vi "Connect temp (SubIV).vi"(8 "Error In":errorcluster, 11 "Loop data In":T2={"Persistent"={"Last file"=path "", "Last user"="", "Users"=[]}, "Temp handle"={"Connected"=FALSE, "Temp ctrl"={"Gain (P)"=0.0, "Reset (I)"=0.0, "Rate (D)"=0.0, "Stabilization rate"=0.0, "Stabilization delta"=0.0, "Type"=enum."Lake Shore 325", "Custom temp ctrl"={"VISA resource name"=""}, "Lakeshore 325"={"VISA name"="", "Loop"=0, "Heater Range"=1, "Heater Resistance"=0, "Sample sensor"=0, "Fast sensor"=0, "Slow sensor"=0}, "Lakeshore 331"={"VISA name"="", "Loop"=1, "Heater Range"=0, "Sample sensor"=0, "Fast sensor"=0, "Slow sensor"=0}, "Lakeshore 332"={"VISA name"="", "Loop"=1, "Heater Range"=0, "Sample sensor"=0, "Fast sensor"=0, "Slow sensor"=0}, "Lakeshore 335"={"VISA name"="", "Loop"=1, "Sample sensor"=0, "Fast sensor"=0, "Slow sensor"=0, "Heater Range"=0, "Output mode"=enum."Off"}, "Lakeshore 336"={"VISA name"="", "Loop"=1, "Output mode"=enum."Off", "Max current"=0.0, "Heater resistance"=0, "Sample sensor"=0, "Slow sensor"=0, "Fast sensor"=1}}}, "Paths"={"Manual"=path "", "Settings"=path "", "Persistent"=path "", "Work dir."=path ""}, "Settings"={"MFIA"={"Address"="", "Use compensation"=TRUE, "Shut down gracefully"=FALSE}, "Temp ctrl"={"Gain (P)"=0.0, "Reset (I)"=0.0, "Rate (D)"=0.0, "Stabilization rate"=0.0, "Stabilization delta"=0.0, "Type"=enum."Lake Shore 325", "Custom temp ctrl"={"VISA resource name"=""}, "Lakeshore 325"={"VISA name"="", "Loop"=0, "Heater Range"=1, "Heater Resistance"=0, "Sample sensor"=0, "Fast sensor"=0, "Slow sensor"=0}, "Lakeshore 331"={"VISA name"="", "Loop"=1, "Heater Range"=0, "Sample sensor"=0, "Fast sensor"=0, "Slow sensor"=0}, "Lakeshore 332"={"VISA name"="", "Loop"=1, "Heater Range"=0, "Sample sensor"=0, "Fast sensor"=0, "Slow sensor"=0}, "Lakeshore 335"={"VISA name"="", "Loop"=1, "Sample sensor"=0, "Fast sensor"=0, "Slow sensor"=0, "Heater Range"=0, "Output mode"=enum."Off"}, "Lakeshore 336"={"VISA name"="", "Loop"=1, "Output mode"=enum."Off", "Max current"=0.0, "Heater resistance"=0, "Sample sensor"=0, "Slow sensor"=0, "Fast sensor"=1}}, "Source-meter"={"Type"=enum."Custom", "Custom source-meter"={"VISA resource name"=""}, "Keithley 2600"={"VISA name"="", "Ignore ID Query"=FALSE, "SMU"=enum."Channel A"}}, "Other"={"Enable OriginLab"=FALSE, "Reader mode"=FALSE, "Auto-save"=FALSE}, "Defaults"={"IV properties"={"T"=0.0, "Vstart"=-0.5, "Vstop"=0.5, "Vpoints"=10.0, "Settling"=0.01, "I limit"=0.1, "Log mapping"=FALSE, "Averaging"=0.0}, "CV properties"={"T"=0.0, "Vstart"=-0.5, "Vstop"=0.5, "Vpoints"=10.0, "Precision"=enum."Normal", "Test signal"=0.01, "Auto I range"=FALSE, "Test frequency"=100000.0, "I range"=-2.0, "V range"=10.0, "Log mapping"=FALSE, "Rel perm"=0.0, "Area"=0.0}, "DLTS properties"={"Tstart"=0.0, "Instant start"=FALSE, "Tstop"=0.0, "T rate"=0.0, "Test signal"=0.0, "Test frequency"=0.0, "Bandwidth"=0.0, "Averaging"=0.0, "Vbias"=0.0, "Vpulse"=0.0, "pulse length"=0.0, "Pulse 2"=FALSE, "Vpulse 2"=0.0, "pulse length 2"=0.0, "I range"=-2.0, "V range"=10.0, "Emission rate"=[], "Sampling rate"=0.0, "Acq. delay"=0.0}, "LDLTS properties"={"T"=0.0, "Test signal"=0.0, "Test frequency"=0.0, "Bandwidth"=0.0, "Averaging"=0.0, "Vbias"=0.0, "Vpulse"=0.0, "pulse length"=0.0, "Pulse 2"=FALSE, "Vpulse 2"=0.0, "pulse length 2"=0.0, "I range"=-2.0, "V range"=10.0, "Sampling rate"=0.0, "Acq. delay"=0.0, "Sampling time"=0.0}}}, "Software version"=0.0, "MFIA handle"={"ziHandle"={"handleValid"=FALSE, "Conn"=0, "Path Prefix"="", "Handle"=0, "Connected"=FALSE, "Clockbase(s)"=0.0}, "Selected device"="", "ziModHandle"={"handleValid"=FALSE, "Conn"=0, "ModHandle"=0, "moduleID"="", "Path Prefix"=""}}, "Source-meter handle"={"Connected"=FALSE, "Source-meter"={"Type"=enum."Keithley 2600", "Custom source-meter"={"VISA resource name"=""}, "Keithley 2600"={"VISA name"="", "Ignore ID Query"=FALSE, "SMU"=enum."Channel A"}}}} {"MFIA handle"."ziModHandle"."ModHandle" format="0x%08x"; "MFIA handle"."ziModHandle"."Conn" format="0x%08x"; "MFIA handle"."ziHandle"."Handle" format="0x%08x"; "MFIA handle"."ziHandle"."Conn" format="0x%08x"; "Settings"."Defaults"."LDLTS properties"."V range" items=["10mV"=0.01, "100mV"=0.1, "1V"=1.0, "10V"=10.0]; "Settings"."Defaults"."LDLTS properties"."I range" items=["100nA"=-7.0, "1µA"=-6.0, "10µA"=-5.0, "100µA"=-4.0, "1mA"=-3.0, "10mA"=-2.0]; "Settings"."Defaults"."DLTS properties"."V range" items=["10mV"=0.01, "100mV"=0.1, "1V"=1.0, "10V"=10.0]; "Settings"."Defaults"."DLTS properties"."I range" items=["10mV"=0.01, "100mV"=0.1, "1V"=1.0, "10V"=10.0]; "Settings"."Defaults"."CV properties"."V range" items=["10mV"=0.01, "100mV"=0.1, "1V"=1.0, "10V"=10.0]; "Settings"."Defaults"."CV properties"."I range" items=["100nA"=-7.0, "1µA"=-6.0, "10µA"=-5.0, "100µA"=-4.0, "1mA"=-3.0, "10mA"=-2.0]; "Settings"."Defaults"."IV properties"."Settling" min=0.0 max=65535.0; "Settings"."Temp ctrl"."Lakeshore 336"."Fast sensor" items=["Sensor A", "Sensor B", "Sensor C", "Sensor D"]; "Settings"."Temp ctrl"."Lakeshore 336"."Slow sensor" items=["Off", "Closed Loop PID", "Zone", "Open Loop", "Monitor Out", "Warmup Supply"]; "Settings"."Temp ctrl"."Lakeshore 336"."Sample sensor" items=["Off", "Low (On)", "Medium", "High"]; "Settings"."Temp ctrl"."Lakeshore 336"."Heater resistance" items=["A", "B"]; "Settings"."Temp ctrl"."Lakeshore 336"."Max current" items=["A", "B"]; "Settings"."Temp ctrl"."Lakeshore 336"."Loop" items=["Loop 1"=1, "Loop 2"=2]; "Settings"."Temp ctrl"."Lakeshore 335"."Heater Range" items=["Off", "Low (On)", "Medium", "High"]; "Settings"."Temp ctrl"."Lakeshore 335"."Slow sensor" items=["A", "B"]; "Settings"."Temp ctrl"."Lakeshore 335"."Fast sensor" items=["25 Ohm"=1, "50 Ohm"=2]; "Settings"."Temp ctrl"."Lakeshore 335"."Sample sensor" items=["Off", "Low (loop 1) or On (loop 2)", "High (loop 1)"]; "Settings"."Temp ctrl"."Lakeshore 335"."Loop" items=["Loop 1"=1, "Loop 2"=2]; "Settings"."Temp ctrl"."Lakeshore 332"."Slow sensor" items=["A", "B"]; "Settings"."Temp ctrl"."Lakeshore 332"."Fast sensor" items=["A", "B"]; "Settings"."Temp ctrl"."Lakeshore 332"."Sample sensor" items=["25 Ohm"=1, "50 Ohm"=2]; "Settings"."Temp ctrl"."Lakeshore 332"."Heater Range" items=["Off", "Low (loop 1) or On (loop 2)", "High (loop 1)"]; "Settings"."Temp ctrl"."Lakeshore 332"."Loop" items=["Loop 1"=1, "Loop 2"=2]; "Settings"."Temp ctrl"."Lakeshore 331"."Slow sensor" items=["A", "B"]; "Settings"."Temp ctrl"."Lakeshore 331"."Fast sensor" items=["A", "B"]; "Settings"."Temp ctrl"."Lakeshore 331"."Sample sensor" items=["25 Ohm"=1, "50 Ohm"=2]; "Settings"."Temp ctrl"."Lakeshore 331"."Heater Range" items=["Off", "Low (loop 1) or On (loop 2)", "High (loop 1)"]; "Settings"."Temp ctrl"."Lakeshore 331"."Loop" items=["Loop 1"=1, "Loop 2"=2]; "Settings"."Temp ctrl"."Lakeshore 325"."Slow sensor" items=["A", "B"]; "Settings"."Temp ctrl"."Lakeshore 325"."Fast sensor" items=["A", "B"]; "Settings"."Temp ctrl"."Lakeshore 325"."Sample sensor" items=["A", "B"]; "Settings"."Temp ctrl"."Lakeshore 325"."Heater Resistance" items=["25 Ohm"=1, "50 Ohm"=2]; "Settings"."Temp ctrl"."Lakeshore 325"."Heater Range" items=["Off", "Low (loop 1) or On (loop 2)", "High (loop 1)"]; "Settings"."Temp ctrl"."Lakeshore 325"."Loop" items=["Loop 1"=1, "Loop 2"=2]; "Temp handle"."Temp ctrl"."Lakeshore 336"."Fast sensor" items=["Sensor A", "Sensor B", "Sensor C", "Sensor D"]; "Temp handle"."Temp ctrl"."Lakeshore 336"."Slow sensor" items=["Off", "Closed Loop PID", "Zone", "Open Loop", "Monitor Out", "Warmup Supply"]; "Temp handle"."Temp ctrl"."Lakeshore 336"."Sample sensor" items=["Off", "Low (On)", "Medium", "High"]; "Temp handle"."Temp ctrl"."Lakeshore 336"."Heater resistance" items=["A", "B"]; "Temp handle"."Temp ctrl"."Lakeshore 336"."Max current" items=["A", "B"]; "Temp handle"."Temp ctrl"."Lakeshore 336"."Loop" items=["Loop 1"=1, "Loop 2"=2]; "Temp handle"."Temp ctrl"."Lakeshore 335"."Heater Range" items=["Off", "Low (On)", "Medium", "High"]; "Temp handle"."Temp ctrl"."Lakeshore 335"."Slow sensor" items=["A", "B"]; "Temp handle"."Temp ctrl"."Lakeshore 335"."Fast sensor" items=["25 Ohm"=1, "50 Ohm"=2]; "Temp handle"."Temp ctrl"."Lakeshore 335"."Sample sensor" items=["Off", "Low (loop 1) or On (loop 2)", "High (loop 1)"]; "Temp handle"."Temp ctrl"."Lakeshore 335"."Loop" items=["Loop 1"=1, "Loop 2"=2]; "Temp handle"."Temp ctrl"."Lakeshore 332"."Slow sensor" items=["A", "B"]; "Temp handle"."Temp ctrl"."Lakeshore 332"."Fast sensor" items=["A", "B"]; "Temp handle"."Temp ctrl"."Lakeshore 332"."Sample sensor" items=["25 Ohm"=1, "50 Ohm"=2]; "Temp handle"."Temp ctrl"."Lakeshore 332"."Heater Range" items=["Off", "Low (loop 1) or On (loop 2)", "High (loop 1)"]; "Temp handle"."Temp ctrl"."Lakeshore 332"."Loop" items=["Loop 1"=1, "Loop 2"=2]; "Temp handle"."Temp ctrl"."Lakeshore 331"."Slow sensor" items=["A", "B"]; "Temp handle"."Temp ctrl"."Lakeshore 331"."Fast sensor" items=["A", "B"]; "Temp handle"."Temp ctrl"."Lakeshore 331"."Sample sensor" items=["25 Ohm"=1, "50 Ohm"=2]; "Temp handle"."Temp ctrl"."Lakeshore 331"."Heater Range" items=["Off", "Low (loop 1) or On (loop 2)", "High (loop 1)"]; "Temp handle"."Temp ctrl"."Lakeshore 331"."Loop" items=["Loop 1"=1, "Loop 2"=2]; "Temp handle"."Temp ctrl"."Lakeshore 325"."Slow sensor" items=["A", "B"]; "Temp handle"."Temp ctrl"."Lakeshore 325"."Fast sensor" items=["A", "B"]; "Temp handle"."Temp ctrl"."Lakeshore 325"."Sample sensor" items=["A", "B"]; "Temp handle"."Temp ctrl"."Lakeshore 325"."Heater Resistance" items=["25 Ohm"=1, "50 Ohm"=2]; "Temp handle"."Temp ctrl"."Lakeshore 325"."Heater Range" items=["Off", "Low (loop 1) or On (loop 2)", "High (loop 1)"]; "Temp handle"."Temp ctrl"."Lakeshore 325"."Loop" items=["Loop 1"=1, "Loop 2"=2]}) -> (0 "Error Out":errorcluster, 2 "Result":T1(ring), 3 "Loop data Out":T2={"Persistent"={"Last file"=path "", "Last user"="", "Users"=[]}, "Temp handle"={"Connected"=FALSE, "Temp ctrl"={"Gain (P)"=0.0, "Reset (I)"=0.0, "Rate (D)"=0.0, "Stabilization rate"=0.0, "Stabilization delta"=0.0, "Type"=enum."Lake Shore 325", "Custom temp ctrl"={"VISA resource name"=""}, "Lakeshore 325"={"VISA name"="", "Loop"=0, "Heater Range"=1, "Heater Resistance"=0, "Sample sensor"=0, "Fast sensor"=0, "Slow sensor"=0}, "Lakeshore 331"={"VISA name"="", "Loop"=1, "Heater Range"=0, "Sample sensor"=0, "Fast sensor"=0, "Slow sensor"=0}, "Lakeshore 332"={"VISA name"="", "Loop"=1, "Heater Range"=0, "Sample sensor"=0, "Fast sensor"=0, "Slow sensor"=0}, "Lakeshore 335"={"VISA name"="", "Loop"=1, "Sample sensor"=0, "Fast sensor"=0, "Slow sensor"=0, "Heater Range"=0, "Output mode"=enum."Off"}, "Lakeshore 336"={"VISA name"="", "Loop"=1, "Output mode"=enum."Off", "Max current"=0.0, "Heater resistance"=0, "Sample sensor"=0, "Slow sensor"=0, "Fast sensor"=1}}}, "Paths"={"Manual"=path "", "Settings"=path "", "Persistent"=path "", "Work dir."=path ""}, "Settings"={"MFIA"={"Address"="", "Use compensation"=TRUE, "Shut down gracefully"=FALSE}, "Temp ctrl"={"Gain (P)"=0.0, "Reset (I)"=0.0, "Rate (D)"=0.0, "Stabilization rate"=0.0, "Stabilization delta"=0.0, "Type"=enum."Lake Shore 325", "Custom temp ctrl"={"VISA resource name"=""}, "Lakeshore 325"={"VISA name"="", "Loop"=0, "Heater Range"=1, "Heater Resistance"=0, "Sample sensor"=0, "Fast sensor"=0, "Slow sensor"=0}, "Lakeshore 331"={"VISA name"="", "Loop"=1, "Heater Range"=0, "Sample sensor"=0, "Fast sensor"=0, "Slow sensor"=0}, "Lakeshore 332"={"VISA name"="", "Loop"=1, "Heater Range"=0, "Sample sensor"=0, "Fast sensor"=0, "Slow sensor"=0}, "Lakeshore 335"={"VISA name"="", "Loop"=1, "Sample sensor"=0, "Fast sensor"=0, "Slow sensor"=0, "Heater Range"=0, "Output mode"=enum."Off"}, "Lakeshore 336"={"VISA name"="", "Loop"=1, "Output mode"=enum."Off", "Max current"=0.0, "Heater resistance"=0, "Sample sensor"=0, "Slow sensor"=0, "Fast sensor"=1}}, "Source-meter"={"Type"=enum."Custom", "Custom source-meter"={"VISA resource name"=""}, "Keithley 2600"={"VISA name"="", "Ignore ID Query"=FALSE, "SMU"=enum."Channel A"}}, "Other"={"Enable OriginLab"=FALSE, "Reader mode"=FALSE, "Auto-save"=FALSE}, "Defaults"={"IV properties"={"T"=0.0, "Vstart"=-0.5, "Vstop"=0.5, "Vpoints"=10.0, "Settling"=0.01, "I limit"=0.1, "Log mapping"=FALSE, "Averaging"=0.0}, "CV properties"={"T"=0.0, "Vstart"=-0.5, "Vstop"=0.5, "Vpoints"=10.0, "Precision"=enum."Normal", "Test signal"=0.01, "Auto I range"=FALSE, "Test frequency"=100000.0, "I range"=-2.0, "V range"=10.0, "Log mapping"=FALSE, "Rel perm"=0.0, "Area"=0.0}, "DLTS properties"={"Tstart"=0.0, "Instant start"=FALSE, "Tstop"=0.0, "T rate"=0.0, "Test signal"=0.0, "Test frequency"=0.0, "Bandwidth"=0.0, "Averaging"=0.0, "Vbias"=0.0, "Vpulse"=0.0, "pulse length"=0.0, "Pulse 2"=FALSE, "Vpulse 2"=0.0, "pulse length 2"=0.0, "I range"=-2.0, "V range"=10.0, "Emission rate"=[], "Sampling rate"=0.0, "Acq. delay"=0.0}, "LDLTS properties"={"T"=0.0, "Test signal"=0.0, "Test frequency"=0.0, "Bandwidth"=0.0, "Averaging"=0.0, "Vbias"=0.0, "Vpulse"=0.0, "pulse length"=0.0, "Pulse 2"=FALSE, "Vpulse 2"=0.0, "pulse length 2"=0.0, "I range"=-2.0, "V range"=10.0, "Sampling rate"=0.0, "Acq. delay"=0.0, "Sampling time"=0.0}}}, "Software version"=0.0, "MFIA handle"={"ziHandle"={"handleValid"=FALSE, "Conn"=0, "Path Prefix"="", "Handle"=0, "Connected"=FALSE, "Clockbase(s)"=0.0}, "Selected device"="", "ziModHandle"={"handleValid"=FALSE, "Conn"=0, "ModHandle"=0, "moduleID"="", "Path Prefix"=""}}, "Source-meter handle"={"Connected"=FALSE, "Source-meter"={"Type"=enum."Keithley 2600", "Custom source-meter"={"VISA resource name"=""}, "Keithley 2600"={"VISA name"="", "Ignore ID Query"=FALSE, "SMU"=enum."Channel A"}}}} {"MFIA handle"."ziModHandle"."ModHandle" format="0x%08x"; "MFIA handle"."ziModHandle"."Conn" format="0x%08x"; "MFIA handle"."ziHandle"."Handle" format="0x%08x"; "MFIA handle"."ziHandle"."Conn" format="0x%08x"; "Settings"."Defaults"."LDLTS properties"."V range" items=["10mV"=0.01, "100mV"=0.1, "1V"=1.0, "10V"=10.0]; "Settings"."Defaults"."LDLTS properties"."I range" items=["100nA"=-7.0, "1µA"=-6.0, "10µA"=-5.0, "100µA"=-4.0, "1mA"=-3.0, "10mA"=-2.0]; "Settings"."Defaults"."DLTS properties"."V range" items=["10mV"=0.01, "100mV"=0.1, "1V"=1.0, "10V"=10.0]; "Settings"."Defaults"."DLTS properties"."I range" items=["10mV"=0.01, "100mV"=0.1, "1V"=1.0, "10V"=10.0]; "Settings"."Defaults"."CV properties"."V range" items=["10mV"=0.01, "100mV"=0.1, "1V"=1.0, "10V"=10.0]; "Settings"."Defaults"."CV properties"."I range" items=["100nA"=-7.0, "1µA"=-6.0, "10µA"=-5.0, "100µA"=-4.0, "1mA"=-3.0, "10mA"=-2.0]; "Settings"."Defaults"."IV properties"."Settling" min=0.0 max=65535.0; "Settings"."Temp ctrl"."Lakeshore 336"."Fast sensor" items=["Sensor A", "Sensor B", "Sensor C", "Sensor D"]; "Settings"."Temp ctrl"."Lakeshore 336"."Slow sensor" items=["Off", "Closed Loop PID", "Zone", "Open Loop", "Monitor Out", "Warmup Supply"]; "Settings"."Temp ctrl"."Lakeshore 336"."Sample sensor" items=["Off", "Low (On)", "Medium", "High"]; "Settings"."Temp ctrl"."Lakeshore 336"."Heater resistance" items=["A", "B"]; "Settings"."Temp ctrl"."Lakeshore 336"."Max current" items=["A", "B"]; "Settings"."Temp ctrl"."Lakeshore 336"."Loop" items=["Loop 1"=1, "Loop 2"=2]; "Settings"."Temp ctrl"."Lakeshore 335"."Heater Range" items=["Off", "Low (On)", "Medium", "High"]; "Settings"."Temp ctrl"."Lakeshore 335"."Slow sensor" items=["A", "B"]; "Settings"."Temp ctrl"."Lakeshore 335"."Fast sensor" items=["25 Ohm"=1, "50 Ohm"=2]; "Settings"."Temp ctrl"."Lakeshore 335"."Sample sensor" items=["Off", "Low (loop 1) or On (loop 2)", "High (loop 1)"]; "Settings"."Temp ctrl"."Lakeshore 335"."Loop" items=["Loop 1"=1, "Loop 2"=2]; "Settings"."Temp ctrl"."Lakeshore 332"."Slow sensor" items=["A", "B"]; "Settings"."Temp ctrl"."Lakeshore 332"."Fast sensor" items=["A", "B"]; "Settings"."Temp ctrl"."Lakeshore 332"."Sample sensor" items=["25 Ohm"=1, "50 Ohm"=2]; "Settings"."Temp ctrl"."Lakeshore 332"."Heater Range" items=["Off", "Low (loop 1) or On (loop 2)", "High (loop 1)"]; "Settings"."Temp ctrl"."Lakeshore 332"."Loop" items=["Loop 1"=1, "Loop 2"=2]; "Settings"."Temp ctrl"."Lakeshore 331"."Slow sensor" items=["A", "B"]; "Settings"."Temp ctrl"."Lakeshore 331"."Fast sensor" items=["A", "B"]; "Settings"."Temp ctrl"."Lakeshore 331"."Sample sensor" items=["25 Ohm"=1, "50 Ohm"=2]; "Settings"."Temp ctrl"."Lakeshore 331"."Heater Range" items=["Off", "Low (loop 1) or On (loop 2)", "High (loop 1)"]; "Settings"."Temp ctrl"."Lakeshore 331"."Loop" items=["Loop 1"=1, "Loop 2"=2]; "Settings"."Temp ctrl"."Lakeshore 325"."Slow sensor" items=["A", "B"]; "Settings"."Temp ctrl"."Lakeshore 325"."Fast sensor" items=["A", "B"]; "Settings"."Temp ctrl"."Lakeshore 325"."Sample sensor" items=["A", "B"]; "Settings"."Temp ctrl"."Lakeshore 325"."Heater Resistance" items=["25 Ohm"=1, "50 Ohm"=2]; "Settings"."Temp ctrl"."Lakeshore 325"."Heater Range" items=["Off", "Low (loop 1) or On (loop 2)", "High (loop 1)"]; "Settings"."Temp ctrl"."Lakeshore 325"."Loop" items=["Loop 1"=1, "Loop 2"=2]; "Temp handle"."Temp ctrl"."Lakeshore 336"."Fast sensor" items=["Sensor A", "Sensor B", "Sensor C", "Sensor D"]; "Temp handle"."Temp ctrl"."Lakeshore 336"."Slow sensor" items=["Off", "Closed Loop PID", "Zone", "Open Loop", "Monitor Out", "Warmup Supply"]; "Temp handle"."Temp ctrl"."Lakeshore 336"."Sample sensor" items=["Off", "Low (On)", "Medium", "High"]; "Temp handle"."Temp ctrl"."Lakeshore 336"."Heater resistance" items=["A", "B"]; "Temp handle"."Temp ctrl"."Lakeshore 336"."Max current" items=["A", "B"]; "Temp handle"."Temp ctrl"."Lakeshore 336"."Loop" items=["Loop 1"=1, "Loop 2"=2]; "Temp handle"."Temp ctrl"."Lakeshore 335"."Heater Range" items=["Off", "Low (On)", "Medium", "High"]; "Temp handle"."Temp ctrl"."Lakeshore 335"."Slow sensor" items=["A", "B"]; "Temp handle"."Temp ctrl"."Lakeshore 335"."Fast sensor" items=["25 Ohm"=1, "50 Ohm"=2]; "Temp handle"."Temp ctrl"."Lakeshore 335"."Sample sensor" items=["Off", "Low (loop 1) or On (loop 2)", "High (loop 1)"]; "Temp handle"."Temp ctrl"."Lakeshore 335"."Loop" items=["Loop 1"=1, "Loop 2"=2]; "Temp handle"."Temp ctrl"."Lakeshore 332"."Slow sensor" items=["A", "B"]; "Temp handle"."Temp ctrl"."Lakeshore 332"."Fast sensor" items=["A", "B"]; "Temp handle"."Temp ctrl"."Lakeshore 332"."Sample sensor" items=["25 Ohm"=1, "50 Ohm"=2]; "Temp handle"."Temp ctrl"."Lakeshore 332"."Heater Range" items=["Off", "Low (loop 1) or On (loop 2)", "High (loop 1)"]; "Temp handle"."Temp ctrl"."Lakeshore 332"."Loop" items=["Loop 1"=1, "Loop 2"=2]; "Temp handle"."Temp ctrl"."Lakeshore 331"."Slow sensor" items=["A", "B"]; "Temp handle"."Temp ctrl"."Lakeshore 331"."Fast sensor" items=["A", "B"]; "Temp handle"."Temp ctrl"."Lakeshore 331"."Sample sensor" items=["25 Ohm"=1, "50 Ohm"=2]; "Temp handle"."Temp ctrl"."Lakeshore 331"."Heater Range" items=["Off", "Low (loop 1) or On (loop 2)", "High (loop 1)"]; "Temp handle"."Temp ctrl"."Lakeshore 331"."Loop" items=["Loop 1"=1, "Loop 2"=2]; "Temp handle"."Temp ctrl"."Lakeshore 325"."Slow sensor" items=["A", "B"]; "Temp handle"."Temp ctrl"."Lakeshore 325"."Fast sensor" items=["A", "B"]; "Temp handle"."Temp ctrl"."Lakeshore 325"."Sample sensor" items=["A", "B"]; "Temp handle"."Temp ctrl"."Lakeshore 325"."Heater Resistance" items=["25 Ohm"=1, "50 Ohm"=2]; "Temp handle"."Temp ctrl"."Lakeshore 325"."Heater Range" items=["Off", "Low (loop 1) or On (loop 2)", "High (loop 1)"]; "Temp handle"."Temp ctrl"."Lakeshore 325"."Loop" items=["Loop 1"=1, "Loop 2"=2]})   [LabVIEW 2019]
doc: "Handles connection to a temperature controller"
uses:
  Type defs/Loop data Type Def.ctl
  Type defs/Persistent Type Def.ctl
  Type defs/Temp handle Type Def.ctl
  Type defs/Temp ctrl Type Def.ctl
  Custom devices/Custom temp ctrl settings.ctl
  Type defs/Paths Type Def.ctl
  Type defs/Settings Type Def.ctl
  Type defs/Imps Type Def.ctl
  Type defs/Source-meter Type Def.ctl
  Custom devices/Custom source-meter settings.ctl
  Type defs/Other settings Type Def.ctl
  Type defs/IV properties Type Def.ctl
  Type defs/CV properties Type Def.ctl
  Type defs/DLTS properties Type Def.ctl
  Type defs/LDLTS properties Type Def.ctl
  Type defs/MFIA handle Type Def.ctl
  <instrlib>/Zurich Instruments LabOne/Public/ziTypeHandle.ctl
  <instrlib>/Zurich Instruments LabOne/Public/Modules/ziTypeModHandle.ctl
  Type defs/Source-meter handle Type Def.ctl
  f0027b96-8a25-4dcd-828b-d9dfff91e735.vi
  <instrlib>/Lake Shore 325/Lake Shore 325.lvlib
  <instrlib>/Lake Shore Cryotronics 332/Lake Shore Cryotronics 332.lvlib
  <instrlib>/Lake Shore Cryotronics 331/Lake Shore Cryotronics 331.lvlib
  <instrlib>/Lake Shore 335/Lake Shore 335.lvlib
  <instrlib>/Lake Shore 336/Lake Shore 336.lvlib
  <instrlib>/Zurich Instruments LabOne/Zurich Instruments LabOne.lvlib
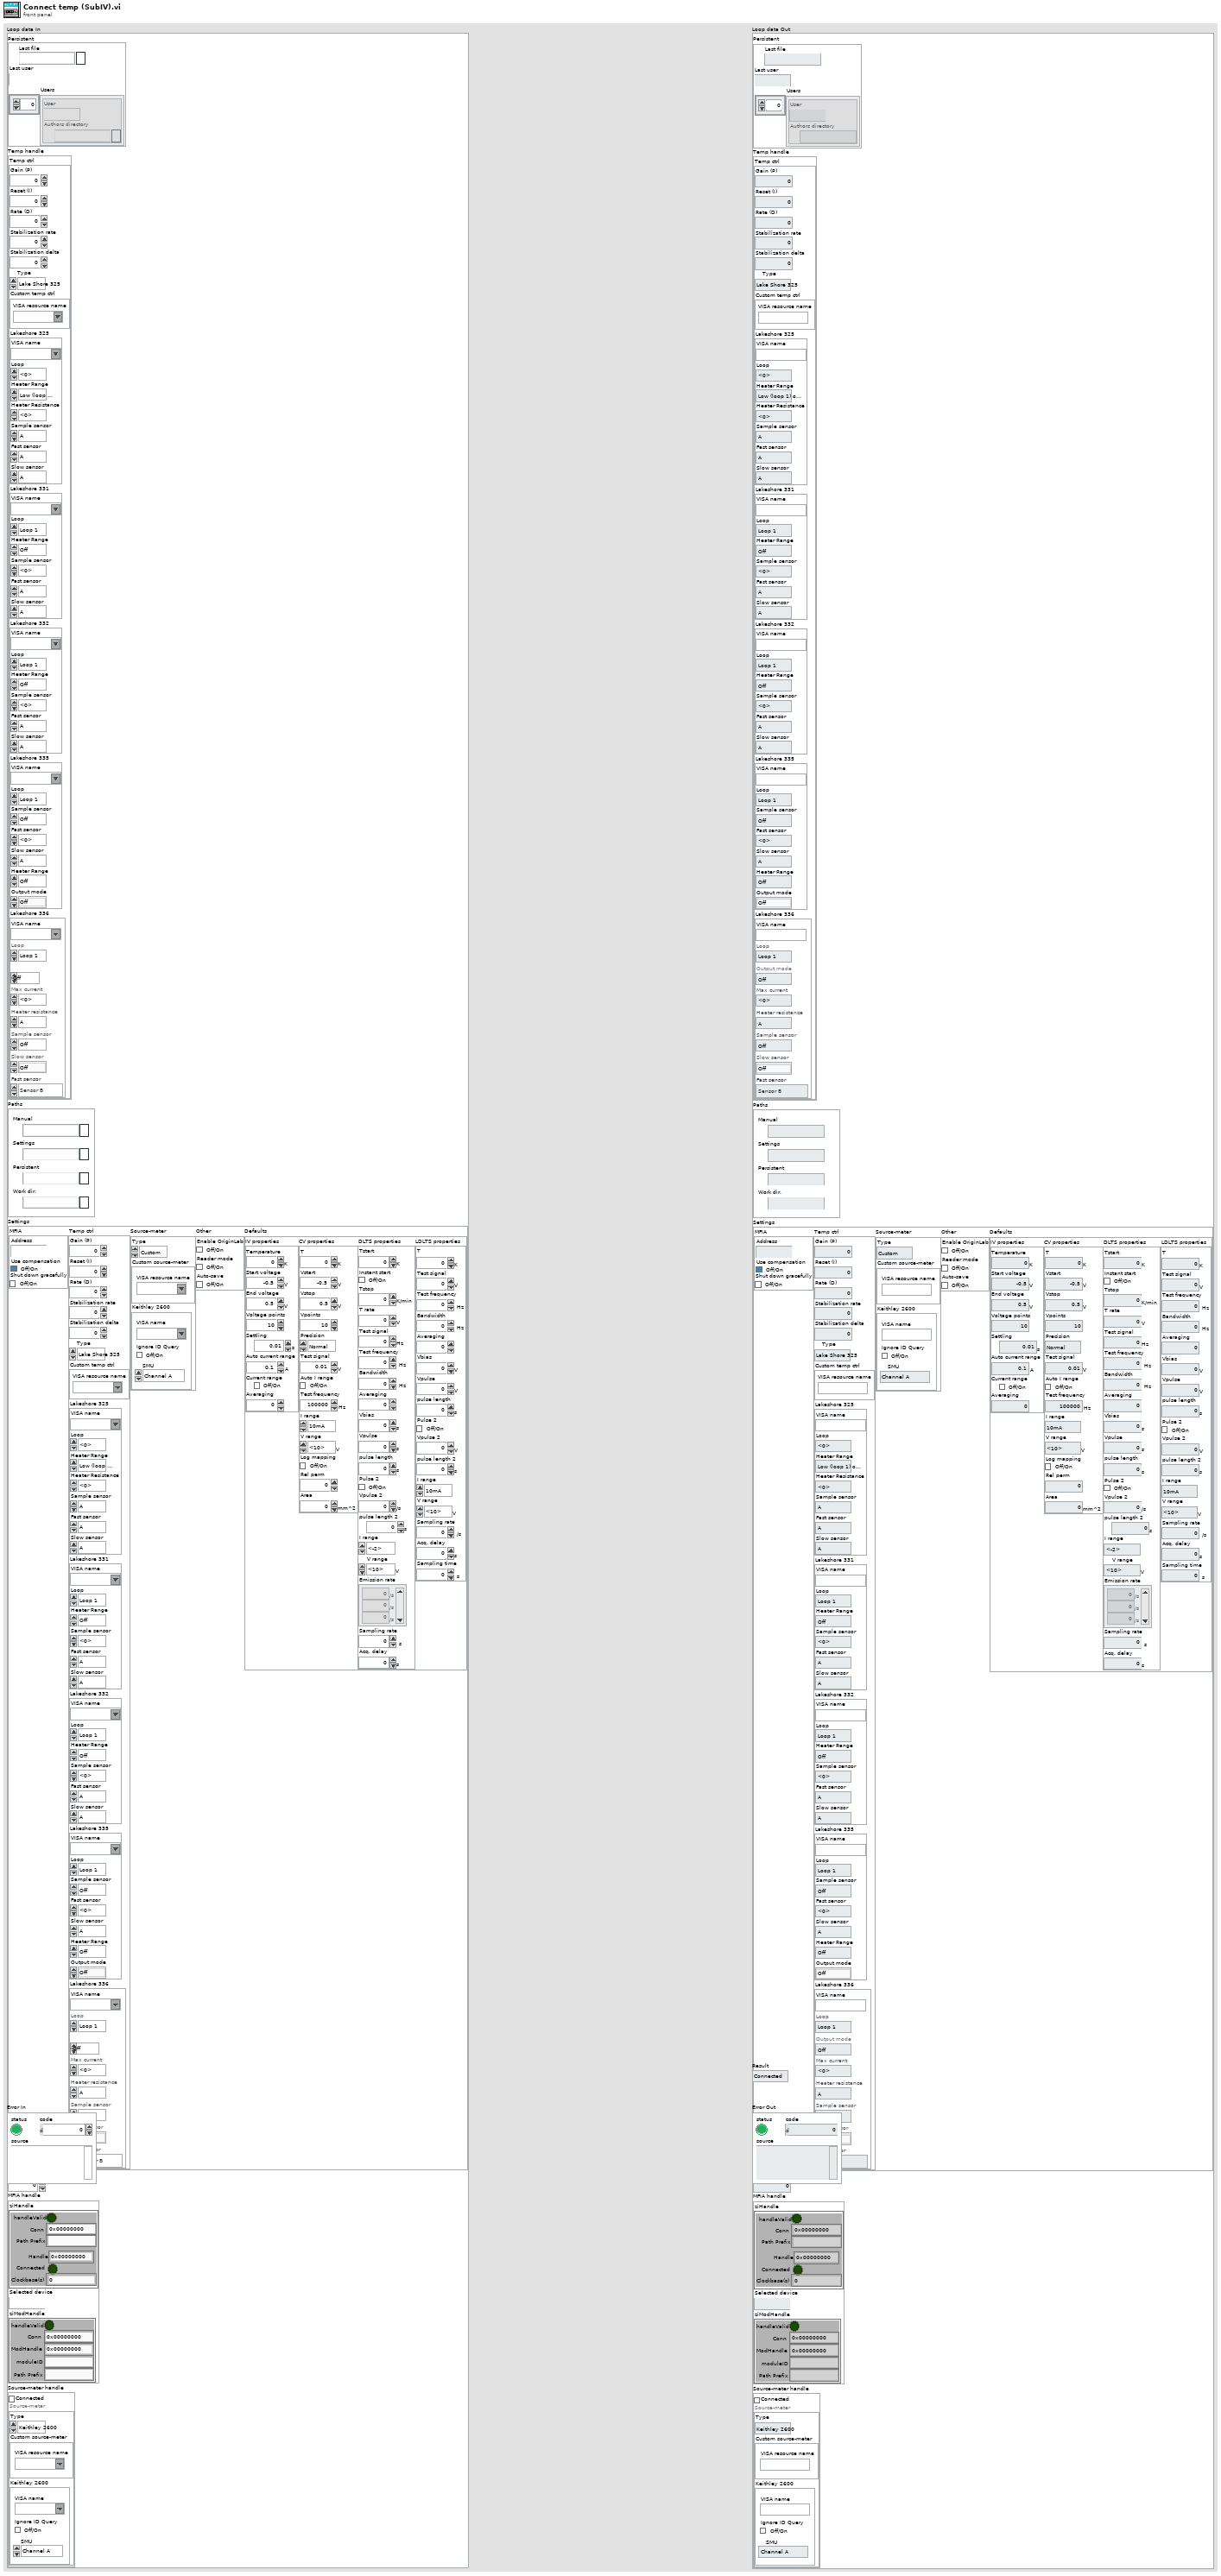
[diagram p1: front panel]
types:
  T1 = enum16{"Connected", "Not connected", "Incorrect settings"}
  T2 = typedef "Loop data Type Def.ctl" = cluster{"Persistent":T3, "Temp handle":T4, "Paths":T7, "Settings":T8, "Software version":dbl, "MFIA handle":T17, "Source-meter handle":T20}
  T3 = typedef "Persistent Type Def.ctl" = cluster{"Last file":path, "Last user":string, "Users":cluster{"User":string, "Authors directory":path}[]}
  T4 = typedef "Temp handle Type Def.ctl" = cluster{"Connected":bool, "Temp ctrl":T5}
  T5 = typedef "Temp ctrl Type Def.ctl" = cluster{"Gain (P)":dbl, "Reset (I)":dbl, "Rate (D)":dbl, "Stabilization rate":dbl, "Stabilization delta":dbl, "Type":enum16{"Custom", "Lake Shore 325", "Lake Shore 331", "Lake Shore 332", "Lake Shore 335", "Lake Shore 336"}, "Custom temp ctrl":T6, "Lakeshore 325":cluster{"VISA name":refnum<visa-resource-name>, "Loop":u16, "Heater Range":u16, "Heater Resistance":u16, "Sample sensor":u16, "Fast sensor":u16, "Slow sensor":u16}, "Lakeshore 331":cluster{"VISA name":refnum<visa-resource-name>, "Loop":u16, "Heater Range":u16, "Sample sensor":u16, "Fast sensor":u16, "Slow sensor":u16}, "Lakeshore 332":cluster{"VISA name":refnum<visa-resource-name>, "Loop":u16, "Heater Range":u16, "Sample sensor":u16, "Fast sensor":u16, "Slow sensor":u16}, "Lakeshore 335":cluster{"VISA name":refnum<visa-resource-name>, "Loop":u16, "Sample sensor":u16, "Fast sensor":u16, "Slow sensor":u16, "Heater Range":u16, "Output mode":enum16{"Off", "Closed Loop PID", "Zone", "Open Loop", "Monitor Out", "Warmup Supply"}}, "Lakeshore 336":cluster{"VISA name":refnum<visa-resource-name>, "Loop":u16, "Output mode":enum16{"Off", "Closed Loop PID", "Zone", "Open Loop"}, "Max current":dbl, "Heater resistance":u16, "Sample sensor":u16, "Slow sensor":u16, "Fast sensor":u16}}
  T6 = typedef "Custom temp ctrl settings.ctl" = cluster{"VISA resource name":refnum<visa-resource-name>}
  T7 = typedef "Paths Type Def.ctl" = cluster{"Manual":path, "Settings":path, "Persistent":path, "Work dir.":path}
  T8 = typedef "Settings Type Def.ctl" = cluster{"MFIA":T9, "Temp ctrl":T5, "Source-meter":T10, "Other":T12, "Defaults":cluster{"IV properties":T13, "CV properties":T14, "DLTS properties":T15, "LDLTS properties":T16}}
  T9 = typedef "Imps Type Def.ctl" = cluster{"Address":string, "Use compensation":bool, "Shut down gracefully":bool}
  T10 = typedef "Source-meter Type Def.ctl" = cluster{"Type":enum16{"Custom", "Keithley 2600"}, "Custom source-meter":T11, "Keithley 2600":cluster{"VISA name":refnum<visa-resource-name>, "Ignore ID Query":bool, "SMU":enum16{"Channel A", "Channel B"}}}
  T11 = typedef "Custom source-meter settings.ctl" = cluster{"VISA resource name":refnum<visa-resource-name>}
  T12 = typedef "Other settings Type Def.ctl" = cluster{"Enable OriginLab":bool, "Reader mode":bool, "Auto-save":bool}
  T13 = typedef "IV properties Type Def.ctl" = cluster{"T":dbl[unit], "Vstart":dbl[unit], "Vstop":dbl[unit], "Vpoints":dbl, "Settling":dbl[unit], "I limit":dbl[unit], "Log mapping":bool, "Averaging":dbl}
  T14 = typedef "CV properties Type Def.ctl" = cluster{"T":dbl[unit], "Vstart":dbl[unit], "Vstop":dbl[unit], "Vpoints":dbl, "Precision":enum16{"Low (Fast)", "Normal", "High (Slow)"}, "Test signal":dbl[unit], "Auto I range":bool, "Test frequency":dbl[unit], "I range":dbl, "V range":dbl[unit], "Log mapping":bool, "Rel perm":dbl, "Area":dbl[unit]}
  T15 = typedef "DLTS properties Type Def.ctl" = cluster{"Tstart":dbl[unit], "Instant start":bool, "Tstop":dbl[unit], "T rate":dbl[unit], "Test signal":dbl[unit], "Test frequency":dbl[unit], "Bandwidth":dbl[unit], "Averaging":dbl, "Vbias":dbl[unit], "Vpulse":dbl[unit], "pulse length":dbl[unit], "Pulse 2":bool, "Vpulse 2":dbl[unit], "pulse length 2":dbl[unit], "I range":dbl, "V range":dbl[unit], "Emission rate":dbl[unit][], "Sampling rate":dbl[unit], "Acq. delay":dbl[unit]}
  T16 = typedef "LDLTS properties Type Def.ctl" = cluster{"T":dbl[unit], "Test signal":dbl[unit], "Test frequency":dbl[unit], "Bandwidth":dbl[unit], "Averaging":dbl, "Vbias":dbl[unit], "Vpulse":dbl[unit], "pulse length":dbl[unit], "Pulse 2":bool, "Vpulse 2":dbl[unit], "pulse length 2":dbl[unit], "I range":dbl, "V range":dbl[unit], "Sampling rate":dbl[unit], "Acq. delay":dbl[unit], "Sampling time":dbl[unit]}
  T17 = typedef "MFIA handle Type Def.ctl" = cluster{"ziHandle":T18, "Selected device":string, "ziModHandle":T19}
  T18 = typedef "Zurich Instruments LabOne.lvlib/ziTypeHandle.ctl" = cluster{"handleValid":bool, "Conn":u64, "Path Prefix":string, "Handle":u64, "Connected":bool, "Clockbase(s)":dbl}
  T19 = typedef "Zurich Instruments LabOne.lvlib/ziTypeModHandle.ctl" = cluster{"handleValid":bool, "Conn":u64, "ModHandle":u64, "moduleID":string, "Path Prefix":string}
  T20 = typedef "Source-meter handle Type Def.ctl" = cluster{"Connected":bool, "Source-meter":T10}
  T21 = enum16{"Custom", "Lake Shore 325", "Lake Shore 331", "Lake Shore 332", "Lake Shore 335", "Lake Shore 336"}
  T22 = enum16{"Off", "Closed Loop PID", "Zone", "Open Loop", "Monitor Out", "Warmup Supply"}
  T23 = enum16{"Off", "Closed Loop PID", "Zone", "Open Loop"}
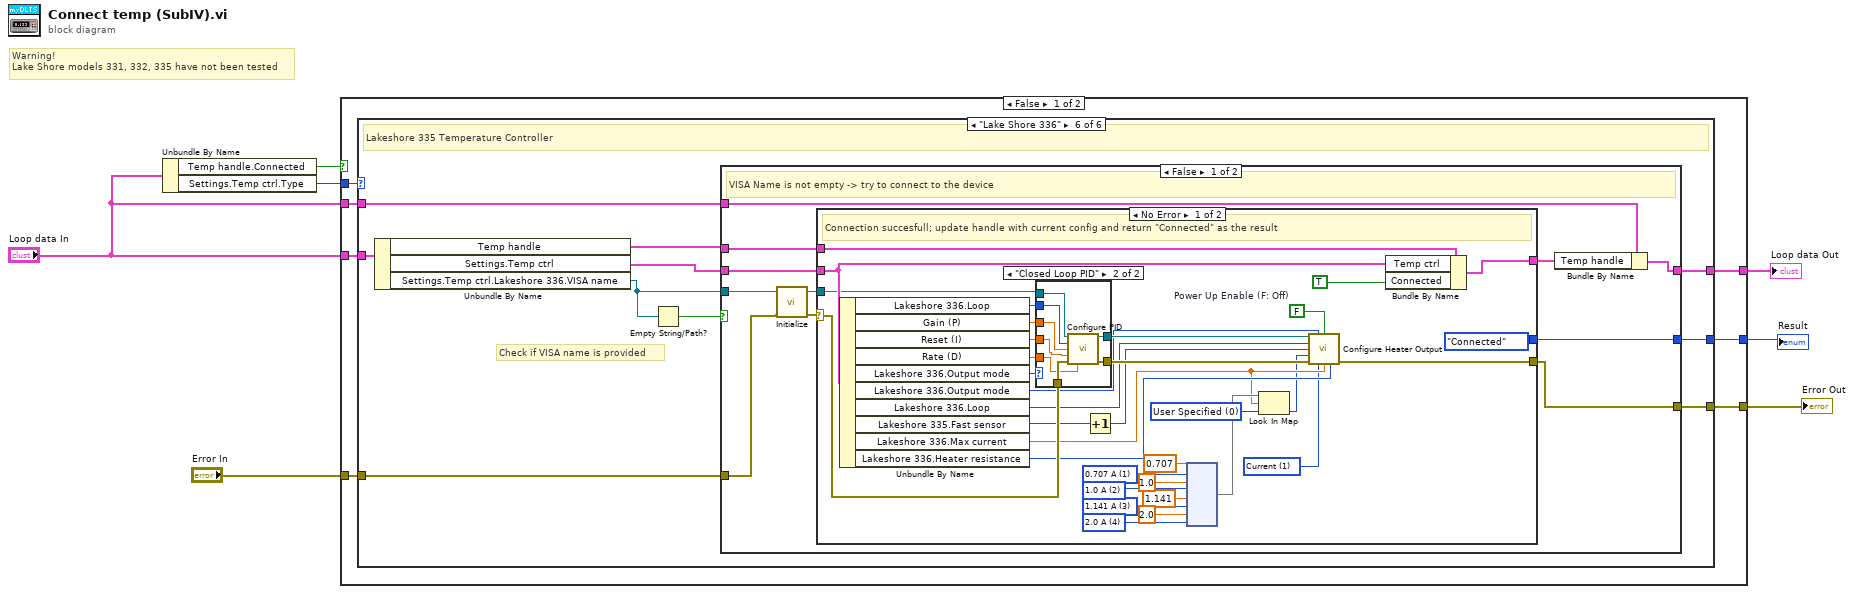
[diagram p0: block diagram]
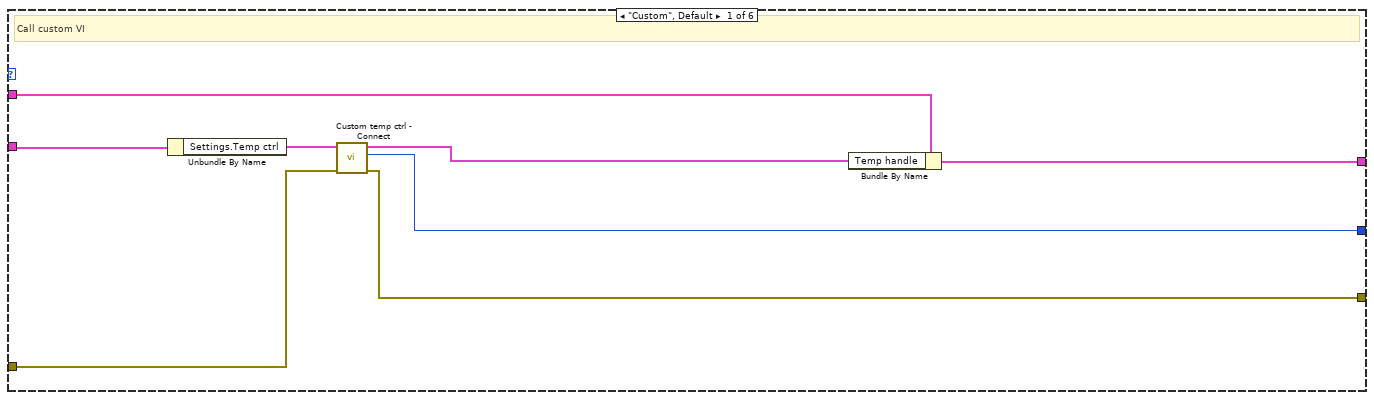
[diagram p2: hidden frame]
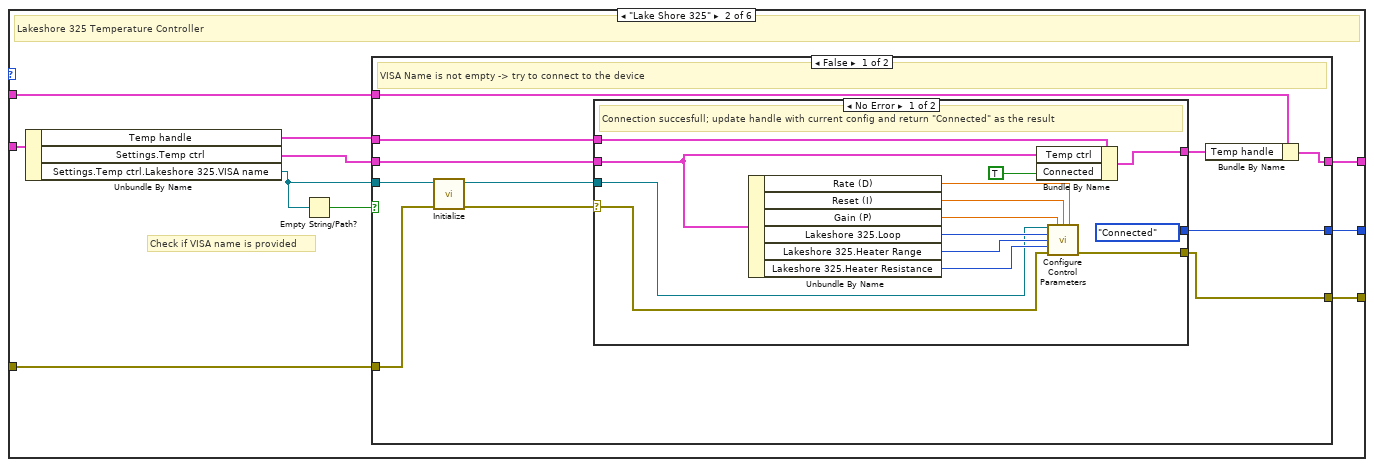
[diagram p3: hidden frame]
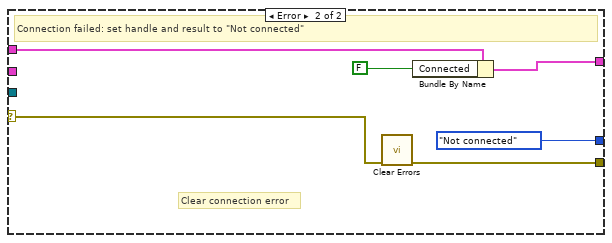
[diagram p4: hidden frame]
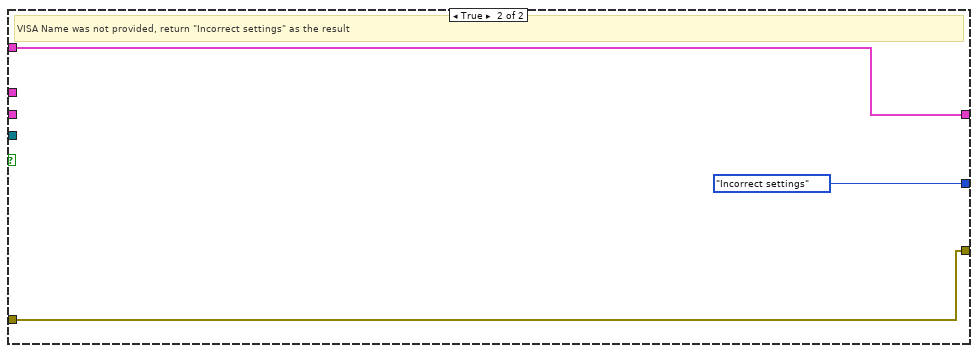
[diagram p5: hidden frame]
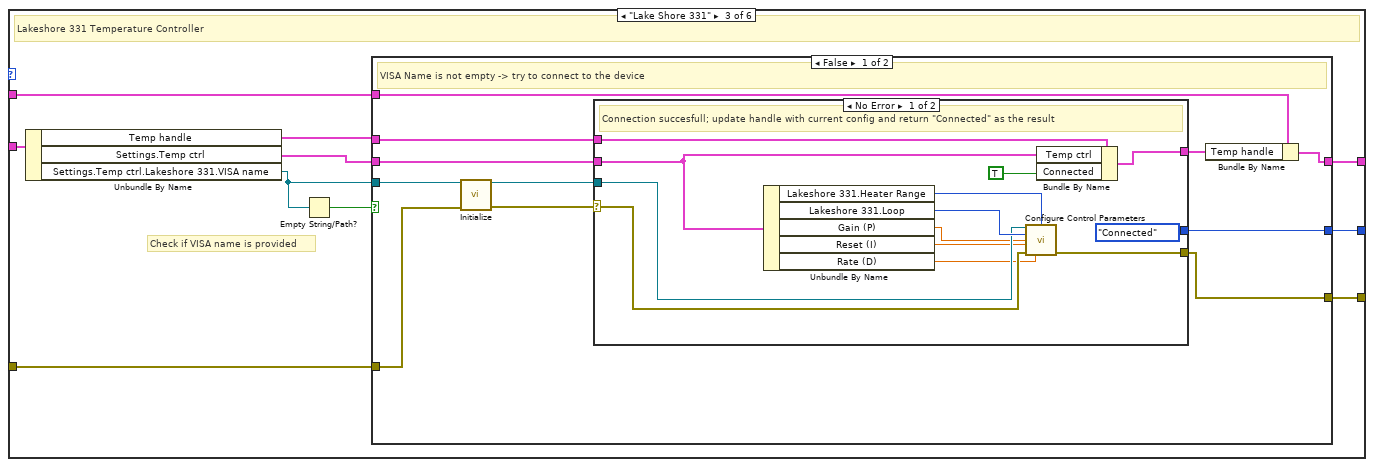
[diagram p6: hidden frame]
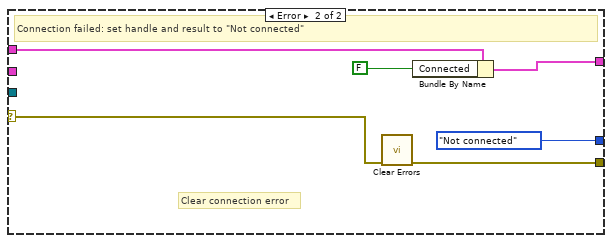
[diagram p7: hidden frame]
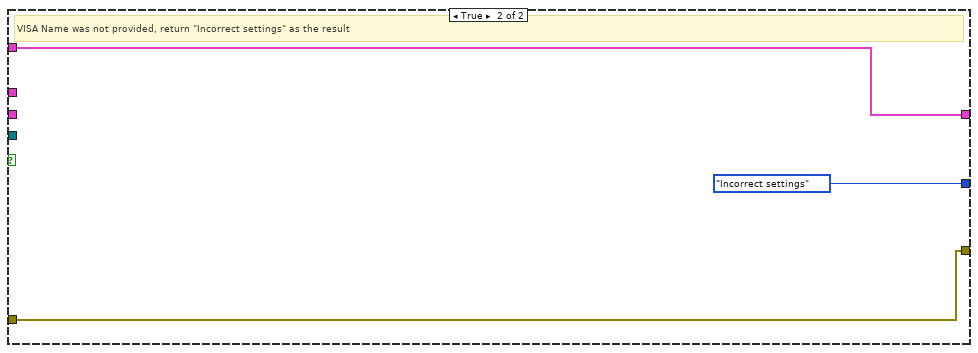
[diagram p8: hidden frame]
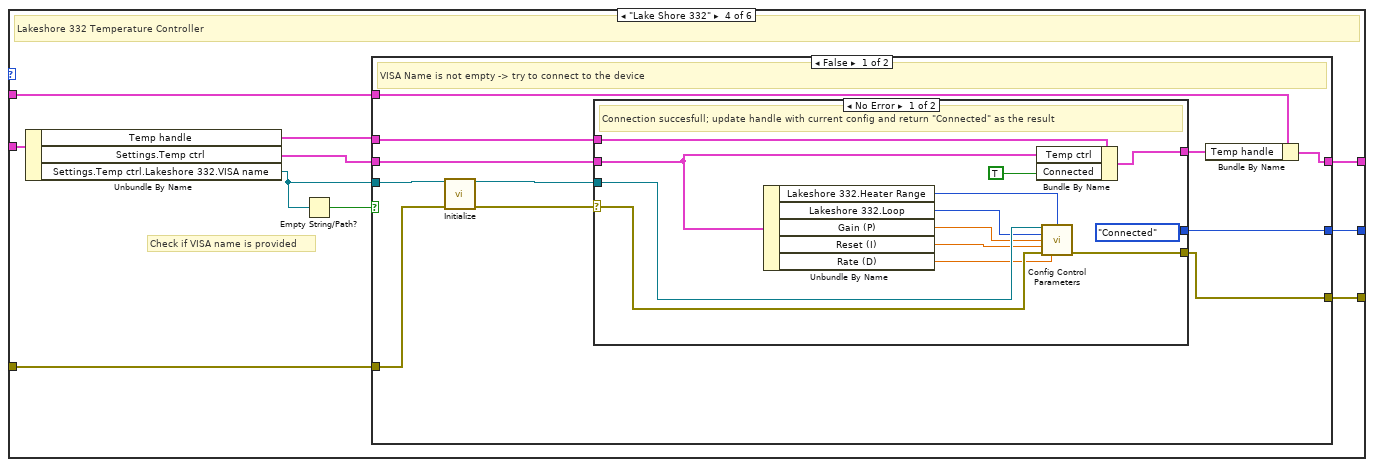
[diagram p9: hidden frame]
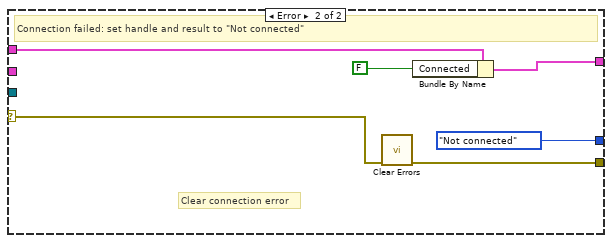
[diagram p10: hidden frame]
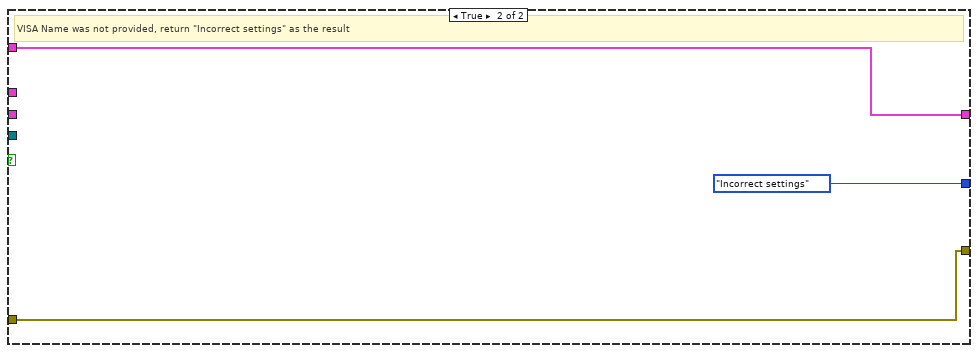
[diagram p11: hidden frame]
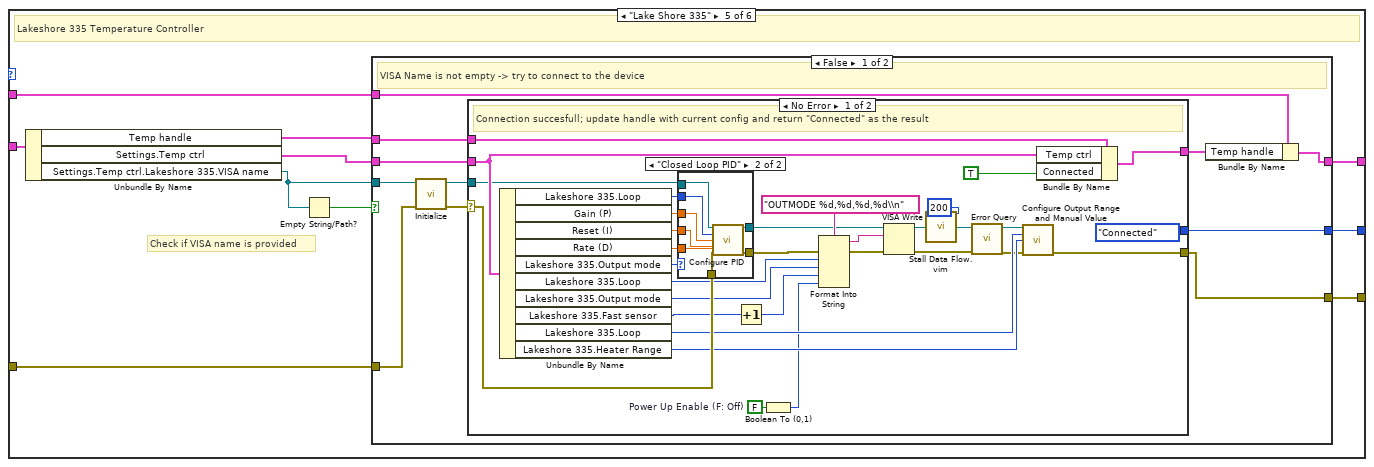
[diagram p12: hidden frame]
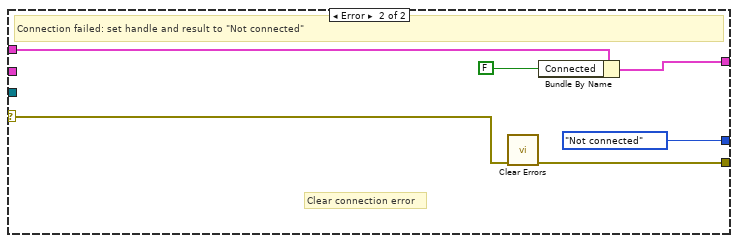
[diagram p14: hidden frame]
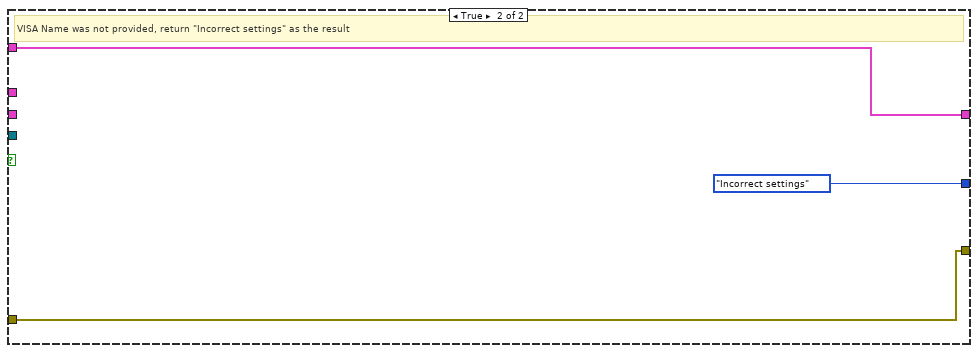
[diagram p15: hidden frame]
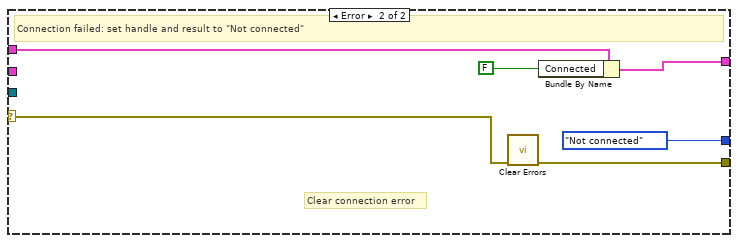
[diagram p17: hidden frame]
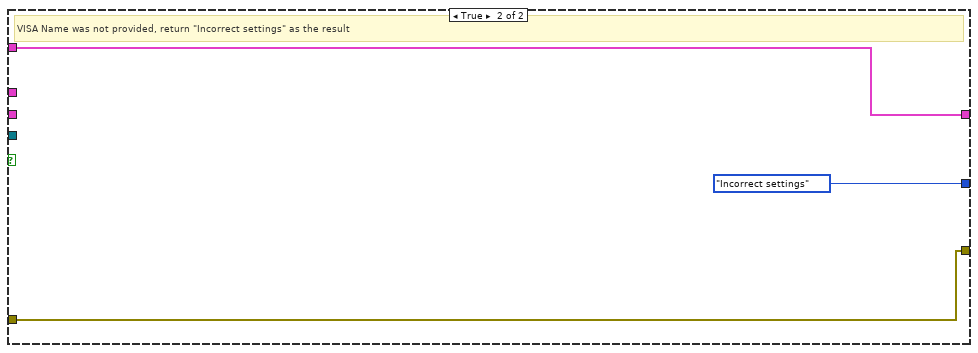
[diagram p18: hidden frame]
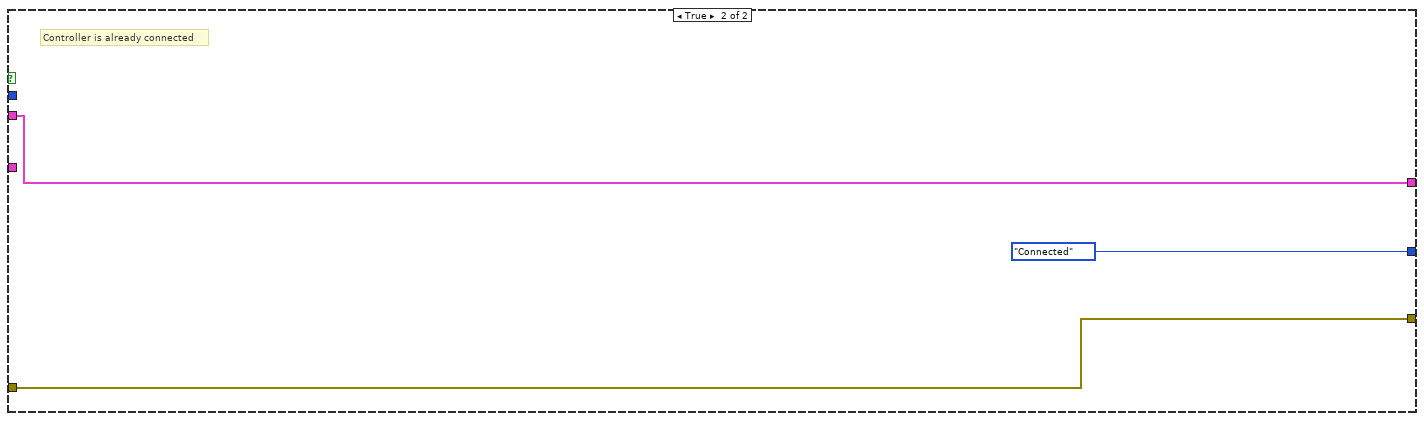
[diagram p19: hidden frame]
diagram:
  # "Warning!\nLake Shore models 331, 332, 335 have not been tested"
  n1 = Unbundle By Name("Loop data In") -> ("Temp handle.Connected"=w3:bool, "Settings.Temp ctrl.Type"=w2:T21)
  n2 = case shown="False" w3 {
    tunnel: [w14 w300] -> w7
    tunnel: [w13 T1."Connected" ("Result")] -> w6
    tunnel: "Error In" -> [w12 w299]
    tunnel: "Loop data In" -> [w11 w300]
    tunnel: [w10 w299] -> w4
    tunnel: w2 -> [w9 _]
    tunnel: "Loop data In" -> [w8 _]
    frame False {
      n3 = case shown="\"Lake Shore 336\"" w9 {
        tunnel: [w20 w30 w74 w117 w160 w232] -> w14
        tunnel: [w17 w32 w76 w119 w162 w234] -> w13
        tunnel: w12 -> [w18 w29 w73 w116 w159 w231]
        tunnel: w11 -> [w21 w28 w72 w115 w158 w230]
        tunnel: [w15 w27 w71 w114 w157 w229] -> w10
        tunnel: w8 -> [w22 w26 w70 w113 w156 w228]
        frame "Custom", Default {
          # "Call custom VI"
          n4 = Unbundle By Name(w22) -> ("Settings.Temp ctrl"=w19:T5)
          n5 = call "Custom temp ctrl - Connect.vi"("Error In"=w18, "Settings.Temp ctrl"=w19) -> ("Error Out"=w15:errorcluster, "Result"=w17:T1, "Temp handle"=w16:T4)  [unwired: 7 in]
          n6 = Bundle By Name(cluster=w21, "Temp handle"=w16) -> (w20:T2)
        }
        frame "Lake Shore 325" {
          # "Check if VISA name is provided"
          # "Lakeshore 325 Temperature Controller"
          n7 = Unbundle By Name(w26) -> ("Temp handle"=w25:T4, "Settings.Temp ctrl"=w23:T5, "Settings.Temp ctrl.Lakeshore 325.VISA name"=w24:refnum<visa-resource-name>)
          n8 = Empty String/Path?(string/path=w24) -> (empty?=w31:bool)
          n9 = case shown="False" w31 {
            tunnel: [w37 T1."Incorrect settings" ("Result")] -> w32
            tunnel: w23 -> [w39 _]
            tunnel: [w34 w65] -> w30
            tunnel: w24 -> [w43 _]
            tunnel: w29 -> [w42 w64]
            tunnel: w25 -> [w38 _]
            tunnel: w28 -> [w36 w65]
            tunnel: [w33 w64] -> w27
            frame False {
              # "VISA Name is not empty -> try to connect to the device"
              n10 = call <instrlib>:"Initialize.vi"("error in (no error)"=w42, "VISA resource name"=w43) -> ("error out"=w41:errorcluster, "VISA resource name out"=w40:refnum<visa-resource-name>)  [unwired: 8 in]
              n11 = case shown="No Error" w41 {
                selector: w41 -> [w51 w60]
                tunnel: w40 -> [w48 _]
                tunnel: [w46 w59] -> w33
                tunnel: w38 -> [w47 w62]
                tunnel: [w49 w61] -> w35
                tunnel: w39 -> [w44 _]
                tunnel: [T1."Connected" ("Result") T1."Not connected" ("Result")] -> w37
                frame No Error {
                  # "Connection succesfull; update handle with current config and return \"Connected\" as the result"
                  n12 = Unbundle By Name(w44) -> ("Rate (D)"=w57:dbl, "Reset (I)"=w56:dbl, "Gain (P)"=w55:dbl, "Lakeshore 325.Loop"=w54:u16, "Lakeshore 325.Heater Range"=w53:u16, "Lakeshore 325.Heater Resistance"=w52:u16)
                  n13 = Bundle By Name(cluster=w47, "Temp ctrl"=w44, "Connected"=TRUE ("Temp handle.Connected")) -> (w49:T4)
                  n14 = call <instrlib>:"Configure Control Parameters.vi"("VISA resource name"=w48, "Gain (P) (0.0)"=w55, "Reset (I) (0.0)"=w56, "Rate (D) (0 %)"=w57, "Loop (1:Loop 1)"=w54, "Heater Range (0:Off)"=w53, "Heater Resistance (1:25 Ohm)"=w52, "error in (no error)"=w51) -> ("error out"=w46:errorcluster)  [unwired: 6 in, 1 out]
                }
                frame Error {
                  # "Clear connection error"
                  # "Connection failed: set handle and result to \"Not connected\""
                  n15 = call <vilib>:"Clear Errors.vi"("error in (no error)"=w60) -> ("error out"=w59:errorcluster)  [unwired: 5 in, 1 out]
                  n16 = Bundle By Name(cluster=w62, "Connected"=FALSE ("Temp handle.Connected")) -> (w61:T4)
                }
              }
              n17 = Bundle By Name(cluster=w36, "Temp handle"=w35) -> (w34:T2)
            }
            frame True {
              # "VISA Name was not provided, return \"Incorrect settings\" as the result"
            }
          }
        }
        frame "Lake Shore 331" {
          # "Check if VISA name is provided"
          # "Lakeshore 331 Temperature Controller"
          n18 = Unbundle By Name(w70) -> ("Temp handle"=w69:T4, "Settings.Temp ctrl"=w67:T5, "Settings.Temp ctrl.Lakeshore 331.VISA name"=w68:refnum<visa-resource-name>)
          n19 = Empty String/Path?(string/path=w68) -> (empty?=w75:bool)
          n20 = case shown="False" w75 {
            tunnel: [w85 T1."Incorrect settings" ("Result")] -> w76
            tunnel: w67 -> [w87 _]
            tunnel: [w82 w108] -> w74
            tunnel: w68 -> [w80 _]
            tunnel: w73 -> [w79 w107]
            tunnel: w69 -> [w86 _]
            tunnel: w72 -> [w84 w108]
            tunnel: [w81 w107] -> w71
            frame False {
              # "VISA Name is not empty -> try to connect to the device"
              n21 = call <instrlib>:"Initialize.vi"("VISA resource name"=w80, "error in (no error)"=w79) -> ("VISA resource name out"=w78:refnum<visa-resource-name>, "error out"=w77:errorcluster)  [unwired: 12 in]
              n22 = case shown="No Error" w77 {
                selector: w77 -> [w92 w103]
                tunnel: w78 -> [w93 _]
                tunnel: [w91 w102] -> w81
                tunnel: w86 -> [w98 w105]
                tunnel: [w99 w104] -> w83
                tunnel: w87 -> [w96 _]
                tunnel: [T1."Connected" ("Result") T1."Not connected" ("Result")] -> w85
                frame No Error {
                  # "Connection succesfull; update handle with current config and return \"Connected\" as the result"
                  n23 = Unbundle By Name(w96) -> ("Lakeshore 331.Heater Range"=w95:u16, "Lakeshore 331.Loop"=w94:u16, "Gain (P)"=w90:dbl, "Reset (I)"=w89:dbl, "Rate (D)"=w88:dbl)
                  n24 = call <instrlib>:"Configure Control Parameters.vi"("VISA resource name"=w93, "Heater Range (0: Off)"=w95, "Loop (0: 1)"=w94, "Gain (P) (0.0)"=w90, "Reset (I) (0.0)"=w89, "error in (no error)"=w92, "Rate (D) (0)"=w88) -> ("error out"=w91:errorcluster)  [unwired: 7 in, 1 out]
                  n25 = Bundle By Name(cluster=w98, "Temp ctrl"=w96, "Connected"=TRUE ("Temp handle.Connected")) -> (w99:T4)
                }
                frame Error {
                  # "Clear connection error"
                  # "Connection failed: set handle and result to \"Not connected\""
                  n26 = call <vilib>:"Clear Errors.vi"("error in (no error)"=w103) -> ("error out"=w102:errorcluster)  [unwired: 5 in, 1 out]
                  n27 = Bundle By Name(cluster=w105, "Connected"=FALSE ("Temp handle.Connected")) -> (w104:T4)
                }
              }
              n28 = Bundle By Name(cluster=w84, "Temp handle"=w83) -> (w82:T2)
            }
            frame True {
              # "VISA Name was not provided, return \"Incorrect settings\" as the result"
            }
          }
        }
        frame "Lake Shore 332" {
          # "Check if VISA name is provided"
          # "Lakeshore 332 Temperature Controller"
          n29 = Unbundle By Name(w113) -> ("Temp handle"=w112:T4, "Settings.Temp ctrl"=w110:T5, "Settings.Temp ctrl.Lakeshore 332.VISA name"=w111:refnum<visa-resource-name>)
          n30 = Empty String/Path?(string/path=w111) -> (empty?=w118:bool)
          n31 = case shown="False" w118 {
            tunnel: [w128 T1."Incorrect settings" ("Result")] -> w119
            tunnel: w110 -> [w130 _]
            tunnel: [w125 w151] -> w117
            tunnel: w111 -> [w123 _]
            tunnel: w116 -> [w122 w150]
            tunnel: w112 -> [w129 _]
            tunnel: w115 -> [w127 w151]
            tunnel: [w124 w150] -> w114
            frame False {
              # "VISA Name is not empty -> try to connect to the device"
              n32 = call <instrlib>:"Initialize.vi"("VISA resource name"=w123, "error in (no error)"=w122) -> ("VISA resource name out"=w121:refnum<visa-resource-name>, "error out"=w120:errorcluster)  [unwired: 12 in]
              n33 = case shown="No Error" w120 {
                selector: w120 -> [w137 w146]
                tunnel: w121 -> [w138 _]
                tunnel: [w132 w145] -> w124
                tunnel: w129 -> [w141 w148]
                tunnel: [w142 w147] -> w126
                tunnel: w130 -> [w139 _]
                tunnel: [T1."Connected" ("Result") T1."Not connected" ("Result")] -> w128
                frame No Error {
                  # "Connection succesfull; update handle with current config and return \"Connected\" as the result"
                  n34 = Unbundle By Name(w139) -> ("Lakeshore 332.Heater Range"=w131:u16, "Lakeshore 332.Loop"=w133:u16, "Gain (P)"=w134:dbl, "Reset (I)"=w135:dbl, "Rate (D)"=w136:dbl)
                  n35 = Bundle By Name(cluster=w141, "Temp ctrl"=w139, "Connected"=TRUE ("Temp handle.Connected")) -> (w142:T4)
                  n36 = call <instrlib>:"Config Control Parameters.vi"("VISA resource name"=w138, "Heater Range (0: Off)"=w131, "Loop (0: 1)"=w133, "Gain (P) (0.0)"=w134, "Reset (I) (0.0)"=w135, "error in (no error)"=w137, "Rate (D) (0)"=w136) -> ("error out"=w132:errorcluster)  [unwired: 7 in, 1 out]
                }
                frame Error {
                  # "Clear connection error"
                  # "Connection failed: set handle and result to \"Not connected\""
                  n37 = call <vilib>:"Clear Errors.vi"("error in (no error)"=w146) -> ("error out"=w145:errorcluster)  [unwired: 5 in, 1 out]
                  n38 = Bundle By Name(cluster=w148, "Connected"=FALSE ("Temp handle.Connected")) -> (w147:T4)
                }
              }
              n39 = Bundle By Name(cluster=w127, "Temp handle"=w126) -> (w125:T2)
            }
            frame True {
              # "VISA Name was not provided, return \"Incorrect settings\" as the result"
            }
          }
        }
        frame "Lake Shore 335" {
          # "Check if VISA name is provided"
          # "Lakeshore 335 Temperature Controller"
          n40 = Unbundle By Name(w156) -> ("Temp handle"=w155:T4, "Settings.Temp ctrl"=w153:T5, "Settings.Temp ctrl.Lakeshore 335.VISA name"=w154:refnum<visa-resource-name>)
          n41 = Empty String/Path?(string/path=w154) -> (empty?=w161:bool)
          n42 = case shown="False" w161 {
            tunnel: [w171 T1."Incorrect settings" ("Result")] -> w162
            tunnel: w153 -> [w173 _]
            tunnel: [w168 w223] -> w160
            tunnel: w154 -> [w166 _]
            tunnel: w159 -> [w165 w222]
            tunnel: w155 -> [w172 _]
            tunnel: w158 -> [w170 w223]
            tunnel: [w167 w222] -> w157
            frame False {
              # "VISA Name is not empty -> try to connect to the device"
              n43 = call <instrlib>:"Initialize.vi"("error in (no error)"=w165, "VISA resource name"=w166) -> ("error out"=w164:errorcluster, "VISA resource name out"=w163:refnum<visa-resource-name>)  [unwired: 8 in]
              n44 = case shown="No Error" w164 {
                selector: w164 -> [w200 w218]
                tunnel: w163 -> [w199 _]
                tunnel: [w194 w217] -> w167
                tunnel: w172 -> [w203 w220]
                tunnel: [w204 w219] -> w169
                tunnel: w173 -> [w201 _]
                tunnel: [T1."Connected" ("Result") T1."Not connected" ("Result")] -> w171
                frame No Error {
                  w182 = FALSE  # Power Up Enable (F: Off)
                  # "Connection succesfull; update handle with current config and return \"Connected\" as the result"
                  n45 = Unbundle By Name(w201) -> ("Lakeshore 335.Loop"=w198:u16, "Gain (P)"=w197:dbl, "Reset (I)"=w196:dbl, "Rate (D)"=w195:dbl, "Lakeshore 335.Output mode"=w174:T22, "Lakeshore 335.Loop"=w177:u16, "Lakeshore 335.Output mode"=w176:T22, "Lakeshore 335.Fast sensor"=w175:u16, "Lakeshore 335.Loop"=w192:u16, "Lakeshore 335.Heater Range"=w193:u16)
                  n46 = case shown="\"Closed Loop PID\"" w174 {
                    tunnel: w200 -> [w206 w215]
                    tunnel: w199 -> [w207 w214]
                    tunnel: w198 -> [_ w213]
                    tunnel: w197 -> [_ w212]
                    tunnel: w196 -> [_ w211]
                    tunnel: w195 -> [_ w210]
                    tunnel: [w207 w209] -> w179
                    tunnel: [w206 w208] -> w178
                    frame "Off", Default {
                    }
                    frame "Closed Loop PID" {
                      n47 = call <instrlib>:"Configure PID.vi"("VISA resource name"=w214, "Output's Control Loop (1:1)"=w213, "Gain (P) (50.0)"=w212, "Reset (I) (20.0)"=w211, "error in (no error)"=w215, "Rate (D) (0.0 %)"=w210) -> ("VISA resource name out"=w209:refnum<visa-resource-name>, "error out"=w208:errorcluster)  [unwired: 8 in]
                    }
                  }
                  n48 = Increment(x=w175) -> (x+1=w191:u16)
                  n49 = Boolean To (0,1)(Boolean=w182) -> (0, 1=w190:i16)
                  n50 = Format Into String(format string="OUTMODE %d,%d,%d,%d\\n", error in=w178, w177, w176, w191, w190) -> (resulting string=w188:string, error out=w189:errorcluster)  [unwired: 1 in]
                  n51 = VISA Write(VISA resource name=w179, write buffer=w188, error in (no error)=w189) -> (VISA resource name out=w185:refnum<visa-resource-name>, error out=w187:errorcluster)  [unwired: 1 out]
                  n52 = call "Stall Data Flow.vim"("value in"=w185, "milliseconds to wait"=u32 200) -> ("value out"=w186:refnum<visa-resource-name>)  [unwired: 1 out]
                  n53 = call <instrlib>:"Error Query.vi"("error in (no error)"=w187, "VISA resource name"=w186) -> ("error out"=w181:errorcluster, "VISA resource name out"=w180:refnum<visa-resource-name>)  [unwired: 7 in, 1 out]
                  n54 = call <instrlib>:"Configure Output Range and Manual Value.vi"("VISA resource name"=w180, "Heater Output (1:1)"=w192, "Range (0:Off)"=w193, "error in (no error)"=w181) -> ("error out"=w194:errorcluster)  [unwired: 10 in, 1 out]
                  n55 = Bundle By Name(cluster=w203, "Temp ctrl"=w201, "Connected"=TRUE ("Temp handle.Connected")) -> (w204:T4)
                }
                frame Error {
                  # "Clear connection error"
                  # "Connection failed: set handle and result to \"Not connected\""
                  n56 = call <vilib>:"Clear Errors.vi"("error in (no error)"=w218) -> ("error out"=w217:errorcluster)  [unwired: 5 in, 1 out]
                  n57 = Bundle By Name(cluster=w220, "Connected"=FALSE ("Temp handle.Connected")) -> (w219:T4)
                }
              }
              n58 = Bundle By Name(cluster=w170, "Temp handle"=w169) -> (w168:T2)
            }
            frame True {
              # "VISA Name was not provided, return \"Incorrect settings\" as the result"
            }
          }
        }
        frame "Lake Shore 336" {
          # "Check if VISA name is provided"
          # "Lakeshore 335 Temperature Controller"
          n59 = Unbundle By Name(w228) -> ("Temp handle"=w227:T4, "Settings.Temp ctrl"=w225:T5, "Settings.Temp ctrl.Lakeshore 336.VISA name"=w226:refnum<visa-resource-name>)
          n60 = Empty String/Path?(string/path=w226) -> (empty?=w233:bool)
          n61 = case shown="False" w233 {
            tunnel: [w243 T1."Incorrect settings" ("Result")] -> w234
            tunnel: w225 -> [w245 _]
            tunnel: [w240 w297] -> w232
            tunnel: w226 -> [w238 _]
            tunnel: w231 -> [w237 w296]
            tunnel: w227 -> [w244 _]
            tunnel: w230 -> [w242 w297]
            tunnel: [w239 w296] -> w229
            frame False {
              # "VISA Name is not empty -> try to connect to the device"
              n62 = call <instrlib>:"Initialize.vi"("error in (no error)"=w237, "VISA resource name"=w238) -> ("error out"=w236:errorcluster, "VISA resource name out"=w235:refnum<visa-resource-name>)  [unwired: 8 in]
              n63 = case shown="No Error" w236 {
                selector: w236 -> [w274 w292]
                tunnel: w235 -> [w273 _]
                tunnel: [w246 w291] -> w239
                tunnel: w244 -> [w277 w294]
                tunnel: [w278 w293] -> w241
                tunnel: w245 -> [w275 _]
                tunnel: [T1."Connected" ("Result") T1."Not connected" ("Result")] -> w243
                frame No Error {
                  w247 = u16 1 items=["Current"=1, "Power"=2] ("Heater Out Display (1:Current)")
                  w248 = u16 0 items=["User Specified", "0.707 A", "1.0 A", "1.141 A", "2.0 A"] ("Max Current (0:User Specified)")
                  w252 = u16 4 items=["User Specified", "0.707 A", "1.0 A", "1.141 A", "2.0 A"] ("Max Current (0:User Specified)")
                  w254 = u16 3 items=["User Specified", "0.707 A", "1.0 A", "1.141 A", "2.0 A"] ("Max Current (0:User Specified)")
                  w256 = u16 2 items=["User Specified", "0.707 A", "1.0 A", "1.141 A", "2.0 A"] ("Max Current (0:User Specified)")
                  w258 = u16 1 items=["User Specified", "0.707 A", "1.0 A", "1.141 A", "2.0 A"] ("Max Current (0:User Specified)")
                  w265 = FALSE  # Power Up Enable (F: Off)
                  # "Connection succesfull; update handle with current config and return \"Connected\" as the result"
                  n64 = Unbundle By Name(w275) -> ("Lakeshore 336.Loop"=w272:u16, "Gain (P)"=w271:dbl, "Reset (I)"=w270:dbl, "Rate (D)"=w269:dbl, "Lakeshore 336.Output mode"=w267:T23, "Lakeshore 336.Output mode"=w263:T23, "Lakeshore 336.Loop"=w262:u16, "Lakeshore 335.Fast sensor"=w268:u16, "Lakeshore 336.Max current"=w250:dbl, "Lakeshore 336.Heater resistance"=w260:u16)
                  n65 = case shown="\"Closed Loop PID\"" w267 {
                    tunnel: w274 -> [w280 w286]
                    tunnel: w273 -> [w281 w287]
                    tunnel: w272 -> [_ w285]
                    tunnel: w271 -> [_ w284]
                    tunnel: w270 -> [_ w282]
                    tunnel: w269 -> [_ w283]
                    tunnel: [w281 w289] -> w266
                    tunnel: [w280 w288] -> w264
                    frame "Off", Default {
                    }
                    frame "Closed Loop PID" {
                      n66 = call <instrlib>:"Configure PID.vi"("VISA resource name"=w287, "Output's Control Loop (1:1)"=w285, "Gain (P) (50.0)"=w284, "Reset (I) (20.0)"=w282, "error in (no error)"=w286, "Rate (D) (0.0 %)"=w283) -> ("VISA resource name out"=w289:refnum<visa-resource-name>, "error out"=w288:errorcluster)  [unwired: 8 in]
                    }
                  }
                  n67 = Increment(x=w268) -> (x+1=w261:u16)
                  n68 = node(0.707, w258, 1.0, w256, 1.141, w254, 2.0, w252) -> (w251:map{dbl, u16})
                  n69 = Look In Map(map=w251, key=w250, default value=w248) -> (value=w249:u16)  [unwired: 1 out]
                  n70 = call <instrlib>:"Configure Heater Output.vi"("VISA resource name"=w266, "Mode (0:Off)"=w263, "Power Up Enable (F: Off)"=w265, "Heater Output (1:1)"=w262, "Input (0:None)"=w261, "Max Current (0:User Specified)"=w249, "error in (no error)"=w264, "Heater Out Display (1:Current)"=w247, "Max User Current (2.000)"=w250, "Heater Resistance (1:25 Ohms)"=w260) -> ("error out"=w246:errorcluster)  [unwired: 4 in, 1 out]
                  n71 = Bundle By Name(cluster=w277, "Temp ctrl"=w275, "Connected"=TRUE ("Temp handle.Connected")) -> (w278:T4)
                }
                frame Error {
                  # "Clear connection error"
                  # "Connection failed: set handle and result to \"Not connected\""
                  n72 = call <vilib>:"Clear Errors.vi"("error in (no error)"=w292) -> ("error out"=w291:errorcluster)  [unwired: 5 in, 1 out]
                  n73 = Bundle By Name(cluster=w294, "Connected"=FALSE ("Temp handle.Connected")) -> (w293:T4)
                }
              }
              n74 = Bundle By Name(cluster=w242, "Temp handle"=w241) -> (w240:T2)
            }
            frame True {
              # "VISA Name was not provided, return \"Incorrect settings\" as the result"
            }
          }
        }
      }
    }
    frame True {
      # "Controller is already connected"
    }
  }
  "Loop data Out" <- w7
  "Error Out" <- w4
  "Result" <- w6
